vi "Dialog-4 - Copy.vi"(8 "error in":errorcluster, 11 "Status":string) -> (0 "error out":errorcluster, 3 "Cancelled?":bool)   [LabVIEW 2018]
doc: "Use this template to create a dialog box with event handling."
panel:
  in  "OK":bool
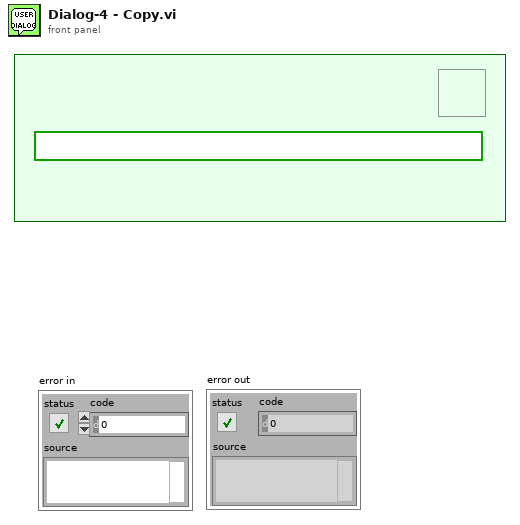
[diagram p1: front panel]
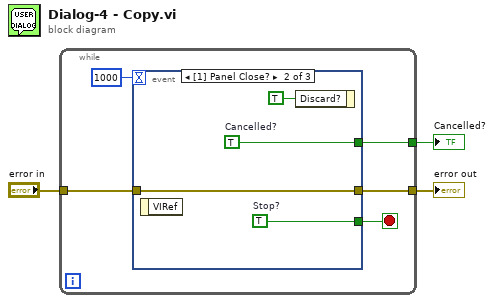
[diagram p0: block diagram]
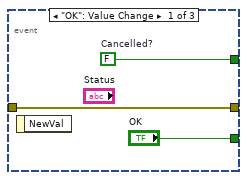
[diagram p2: hidden frame]
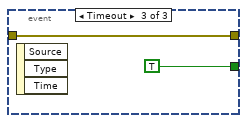
[diagram p3: hidden frame]
diagram:
  n1 = while {
    tunnel: [w7] -> w3
    tunnel: "error in" -> [w5]
    tunnel: [w4] -> w1
    stop <- w8 stop-if-true
    n2 = event shown="[1] Panel Close?" {
      selector: _ -> [_ _ _]
      dyn-events: _ -> [_ _ _]
      timeout: 1000 -> [_ _ _]
      tunnel: ["OK" w14 TRUE ("Stop?")] -> w8
      tunnel: [w11 w13 _] -> w7
      tunnel: w5 -> [w9 w12 w16]
      tunnel: [w9 w12 w16] -> w4
      event "OK": Value Change {
        w11 = FALSE  # Cancelled?
        n3 = event-data() -> ()  [unwired: 1 in, 1 out]
      }
      event Panel Close? {
        w13 = TRUE  # Cancelled?
        w14 = TRUE  # Stop?
        n4 = event-data() -> ()  [unwired: 1 in, 1 out]
        n5 = event-data("Discard?"=TRUE) -> ()  [unwired: 1 in, 1 out]
      }
      event Timeout {
        n6 = event-data() -> ()  [unwired: 1 in, 3 out]
      }
    }
  }
  "Cancelled?" <- w3
  "error out" <- w1
